vi "加标回收停止对话框.vi"() -> ()   [LabVIEW 2016, in "质控单元V4.lvlib"]
panel:
  in  "取消":bool
  in  "确认":bool
  in  "CODCr":bool caption="启用"
  in  "CODMn":bool caption="启用"
  in  "总氮":bool caption="启用"
  in  "总磷":bool caption="启用"
  in  "氨氮":bool caption="启用"
  # "请选择要停止的参数"
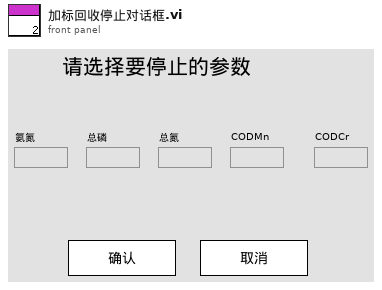
[diagram p1: front panel]
types:
  T1 = cluster{"氨氮":bool, "总磷":bool, "总氮":bool, "CODMn":bool, "CODCr":bool, "氨氮总磷":bool, "总磷总氮":bool}
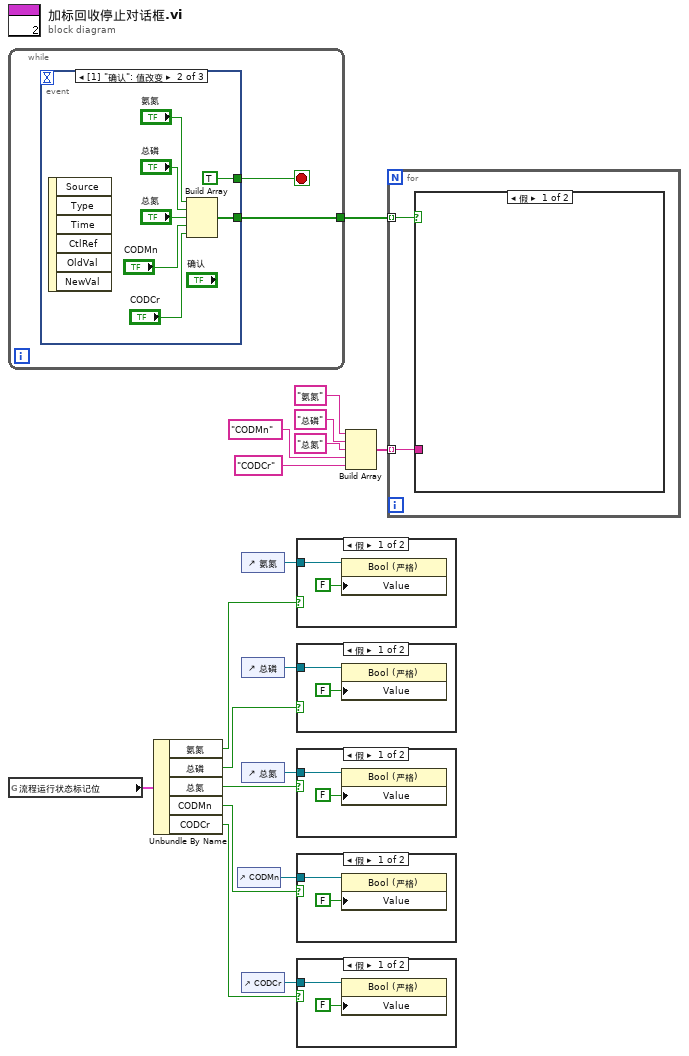
[diagram p0: block diagram]
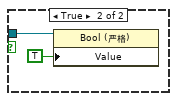
[diagram p2: hidden frame]
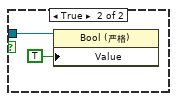
[diagram p3: hidden frame]
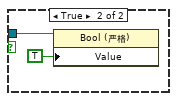
[diagram p4: hidden frame]
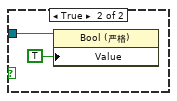
[diagram p5: hidden frame]
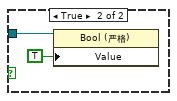
[diagram p6: hidden frame]
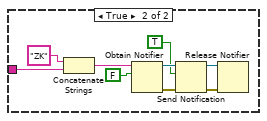
[diagram p7: hidden frame]
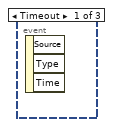
[diagram p8: hidden frame]
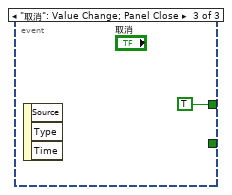
[diagram p9: hidden frame]
diagram:
  n1 = while {
    tunnel: [w19] -> w12
    stop <- w20 stop-if-true
    n2 = event shown="[1] \"确认\": 值改变" {
      selector: _ -> [_ _ _]
      dyn-events: _ -> [_ _ _]
      timeout: _ -> [_ _ _]
      tunnel: [_ TRUE TRUE] -> w20
      tunnel: [_ w21 _] -> w19
      event Timeout {
        n3 = event-data() -> ()  [unwired: 1 in, 3 out]
      }
      event "确认": Value Change {
        n4 = event-data() -> ()  [unwired: 1 in, 6 out]
        n5 = Build Array("氨氮", "总磷", "总氮", "CODMn", "CODCr") -> (w21:bool[])
      }
      event "取消": Value Change; Panel Close {
        n6 = event-data() -> ()  [unwired: 1 in, 3 out]
      }
    }
  }
  n7 = global read "ZK非断电保存全局变量.vi" "流程运行状态标记位"() -> (w11:T1)
  n8 = Unbundle By Name(w11) -> ("氨氮"=w10:bool, "总磷"=w9:bool, "总氮"=w8:bool, "CODMn"=w7:bool, "CODCr"=w6:bool)
  n9 = control-ref of="CODMn"() -> (w2:refnum<vi>)
  n10 = control-ref of="氨氮"() -> (w5:refnum<vi>)
  n11 = control-ref of="总磷"() -> (w4:refnum<vi>)
  n12 = control-ref of="总氮"() -> (w3:refnum<vi>)
  n13 = control-ref of="CODCr"() -> (w1:refnum<vi>)
  n14 = case shown="假" w10 {
    tunnel: w5 -> [w30 w32]
    frame False {
      n15 = property class="Bool (严格)"(reference=w30, "Value"=FALSE ("值")) -> ()  [unwired: 1 in, 2 out]
    }
    frame True {
      n16 = property class="Bool (严格)"(reference=w32, "Value"=TRUE ("值")) -> ()  [unwired: 1 in, 2 out]
    }
  }
  n17 = case shown="假" w9 {
    tunnel: w4 -> [w34 w36]
    frame False {
      n18 = property class="Bool (严格)"(reference=w34, "Value"=FALSE ("值")) -> ()  [unwired: 1 in, 2 out]
    }
    frame True {
      n19 = property class="Bool (严格)"(reference=w36, "Value"=TRUE ("值")) -> ()  [unwired: 1 in, 2 out]
    }
  }
  n20 = case shown="假" w8 {
    tunnel: w3 -> [w38 w40]
    frame False {
      n21 = property class="Bool (严格)"(reference=w38, "Value"=FALSE ("值")) -> ()  [unwired: 1 in, 2 out]
    }
    frame True {
      n22 = property class="Bool (严格)"(reference=w40, "Value"=TRUE ("值")) -> ()  [unwired: 1 in, 2 out]
    }
  }
  n23 = case shown="假" w7 {
    tunnel: w2 -> [w42 w44]
    frame False {
      n24 = property class="Bool (严格)"(reference=w42, "Value"=FALSE ("值")) -> ()  [unwired: 1 in, 2 out]
    }
    frame True {
      n25 = property class="Bool (严格)"(reference=w44, "Value"=TRUE ("值")) -> ()  [unwired: 1 in, 2 out]
    }
  }
  n26 = case shown="假" w6 {
    tunnel: w1 -> [w46 w48]
    frame False {
      n27 = property class="Bool (严格)"(reference=w46, "Value"=FALSE ("值")) -> ()  [unwired: 1 in, 2 out]
    }
    frame True {
      n28 = property class="Bool (严格)"(reference=w48, "Value"=TRUE ("值")) -> ()  [unwired: 1 in, 2 out]
    }
  }
  n29 = Build Array("氨氮", "总磷", "总氮", "CODMn", "CODCr") -> (w13:string[])
  n30 = for {
    tunnel: w13 -> [w50] mode=indexing
    tunnel: w12 -> [w49] mode=indexing
    n31 = case shown="假" w49 {
      tunnel: w50 -> [_ w51]
      frame False {
      }
      frame True {
        n32 = Concatenate Strings("ZK" ("名称（未命名）"), w51) -> (w57:string)
        n33 = Obtain Notifier(name (unnamed)=w57, notification data type=FALSE) -> (notifier out=w56:refnum<notifier>, error out=w55:errorcluster)  [unwired: 2 in, 1 out]
        n34 = Send Notification(notification=TRUE ("通知"), notifier=w56, error in (no error)=w55) -> (notifier out=w54:refnum<notifier>, error out=w53:errorcluster)
        n35 = Release Notifier(notifier=w54, error in (no error)=w53) -> ()  [unwired: 1 in, 3 out]
      }
    }
  }
